vi "Dist.Lane(SubVI).vi"(1 "x0":dbl, 2 "y0":dbl, 3 "x2":dbl, 4 "x1":dbl, 5 "y2":dbl, 6 "y1":dbl) -> (0 "Dist.Lane":dbl)   [LabVIEW 2024]
panel:
  # "p0"
  # "p2"
  # "p1"
  # "Left : (-)\nRight : (+)"
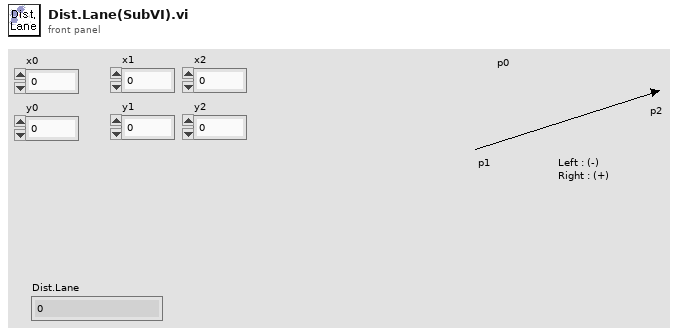
[diagram p1: front panel]
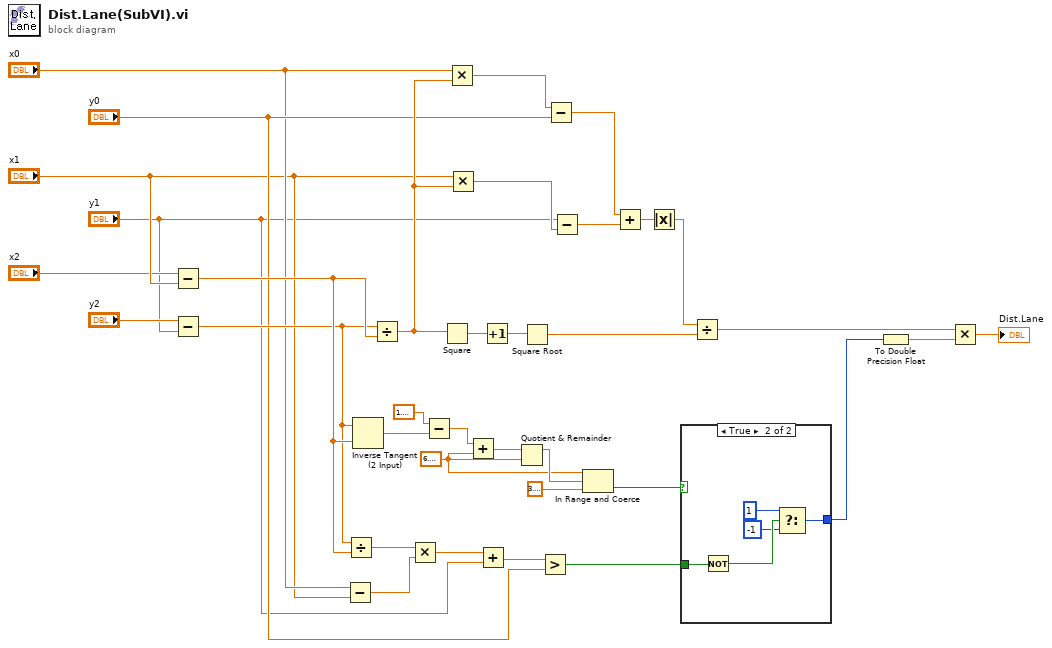
[diagram p0: block diagram]
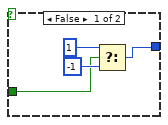
[diagram p2: hidden frame]
diagram:
  w20 = 6.283185307179586
  n1 = Subtract(x="x2", y="x1") -> (x-y=w18:dbl)
  n2 = Subtract(x="y2", y="y1") -> (x-y=w17:dbl)
  n3 = Subtract(x="x0", y="x1") -> (x-y=w15:dbl)
  n4 = Divide(x=w17, y=w18) -> (x/y=w16:dbl)
  n5 = Inverse Tangent (2 Input)(1:w18, 2:w17) -> (0:w25:dbl)
  n6 = Divide(x=w17, y=w18) -> (x/y=w31:dbl)
  n7 = Multiply(x=w16, y=w15) -> (x*y=w14:dbl)
  n8 = Subtract(x=1.5707963267948966, y=w25) -> (x-y=w23:dbl)
  n9 = Square(x=w31) -> (x^2=w35:dbl)
  n10 = Multiply(x="x0", y=w31) -> (x*y=w32:dbl)
  n11 = Multiply(x="x1", y=w31) -> (x*y=w30:dbl)
  n12 = Add(x=w23, y=w20) -> (x+y=w22:dbl)
  n13 = Add(x=w14, y="y1") -> (x+y=w13:dbl)
  n14 = Increment(x=w35) -> (x+1=w34:dbl)
  n15 = Quotient & Remainder(x=w22, y=w20) -> (x-y*floor(x/y)=w21:dbl)  [unwired: 1 out]
  n16 = Square Root(x=w34) -> (sqrt(x)=w33:dbl)
  n17 = Greater?(x=w13, y="y0") -> (0:w11:bool)
  n18 = Subtract(x=w32, y="y0") -> (x-y=w29:dbl)
  n19 = Subtract(x="y1", y=w30) -> (x-y=w28:dbl)
  n20 = In Range and Coerce(upper limit=w20, x=w21, lower limit=3.141592653589793) -> (In Range?=w12:bool)  [unwired: 1 out]
  n21 = Add(x=w29, y=w28) -> (x+y=w27:dbl)
  n22 = Absolute Value(x=w27) -> (abs(x)=w26:dbl)
  n23 = case shown="True" w12 {
    tunnel: w11 -> [w36 w41]
    tunnel: [w37 w40] -> w9
    frame False {
      n24 = Select(t=1, s=w36, f=-1) -> (s? t:f=w37:i32)
    }
    frame True {
      n25 = Not(x=w41) -> (.not. x?=w44:bool)
      n26 = Select(t=1, s=w44, f=-1) -> (s? t:f=w40:i32)
    }
  }
  n27 = Divide(x=w26, y=w33) -> (x/y=w10:dbl)
  n28 = To Double Precision Float(number=w9) -> (double precision float=w1:dbl)
  n29 = Multiply(x=w10, y=w1) -> (x*y=→"Dist.Lane":dbl)
